vi "Test Basic Forms.vi"() -> ()   [LabVIEW 2020]
uses:
  HTTP Server/Server/Server.lvclass
  HTTP Server/RequestTraceLog/RequestTraceLog.lvclass
  HTTP Server/StandardFileServe/StandardFileServe.lvclass
  C:/dev/IlluminatedG/lv-http-server/HTTP Server/Controller/Controller.lvclass
  C:/dev/IlluminatedG/lv-http-server/HTTP Server/Handler/Handler.lvclass
  C:/dev/IlluminatedG/lv-http-server/HTTP Server/StandardFileServe/StandardFileServe.lvclass
  HTTP Server/Processing Step.ctl
  HTTP Server/HTTP Server.lvlib
  HTTP Server/Trace Item.ctl
  HTTP Server/Trace Log.ctl
panel:
  in  "Debug":bool=TRUE
  out "error out":errorcluster
  in  "Port":u16=36987
  in  "Refresh Traces":bool
  out "Traces":T1[](array[typedef]) {"Items"."Time" format="%.6f"}
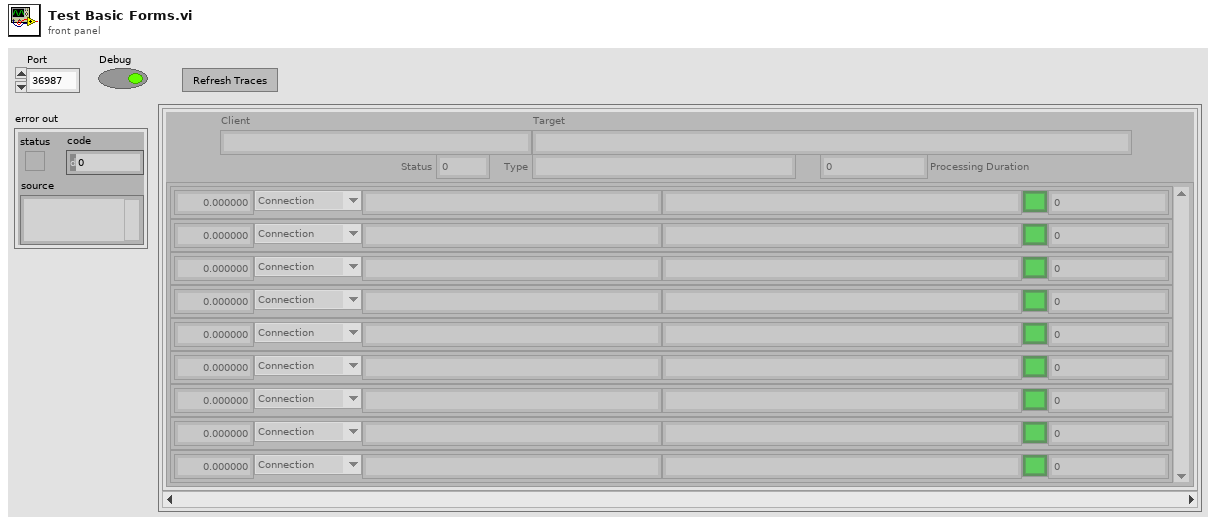
[diagram p1: front panel]
types:
  T1 = typedef "HTTP Server.lvlib/Trace Log.ctl" = cluster{"Client":string, "Target":string, "Status":u16, "Type":string, "Processing Duration":dbl, "Items":T2[]}
  T2 = typedef "HTTP Server.lvlib/Trace Item.ctl" = cluster{"Time":dbl, "Processing Step":T3, "Class":string, "Info":string, "Status":bool, "Code":i32}
  T3 = typedef "HTTP Server.lvlib/Processing Step.ctl" = enum16{"Connection", "Request", "Routing", "Controller Init", "Controller", "Response", "Complete", "Exception"}
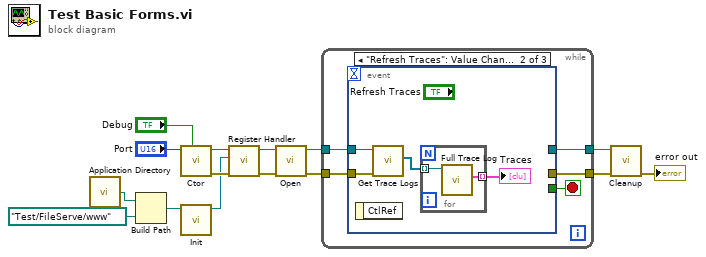
[diagram p0: block diagram]
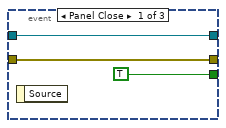
[diagram p2: hidden frame]
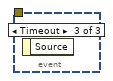
[diagram p3: hidden frame]
diagram:
  n1 = call <vilib>:"Application Directory.vi"() -> ("Application Directory"=w9:path)
  n2 = Build Path(base path=w9, name or relative path=path "Test/FileServe/www") -> (appended path=w7:path)
  n3 = call "Ctor.vi"("Debug (F)"="Debug", "Port (8080)"="Port") -> ("error out"=w3:errorcluster, "Server out"=w5:refnum<class "Server.lvclass">)  [unwired: 8 in]
  n4 = call "Init.vi"("Public Root"=w7) -> ("StandardFileServe out"=w1:refnum<class "StandardFileServe.lvclass">)  [unwired: 9 in, 1 out]
  n5 = call "Register Handler.vi"("error in (no error)"=w3, "Handler"=w1, "Server in"=w5) -> ("error out"=w2:errorcluster, "Server out"=w4:refnum<class "Server.lvclass">)  [unwired: 7 in]
  n6 = call "Open.vi"("error in (no error)"=w2, "Server in"=w4) -> ("error out"=w13:errorcluster, "Server out"=w14:refnum<class "Server.lvclass">)  [unwired: 8 in]
  n7 = while {
    tunnel: w14 -> [w18]
    tunnel: w13 -> [w19]
    tunnel: [w17] -> w12
    tunnel: [w16] -> w11
    stop <- w20 stop-if-true
    n8 = event shown="[1] \"Refresh Traces\": Value Change" {
      selector: _ -> [_ _ _]
      dyn-events: _ -> [_ _ _]
      timeout: _ -> [_ _ _]
      tunnel: [TRUE ("Discard?") _ _] -> w20
      tunnel: w19 -> [w21 w26 _]
      tunnel: w18 -> [w22 w27 _]
      tunnel: [w22 _ _] -> w17
      tunnel: [w21 _ _] -> w16
      event Panel Close {
        n9 = event-data() -> ()  [unwired: 1 in, 1 out]
      }
      event "Refresh Traces": Value Change {
        n10 = event-data() -> ()  [unwired: 1 in, 1 out]
        n11 = call "Get Trace Logs.vi"("error in (no error)"=w26, "Server in"=w27) -> ("Trace Logs"=w25:refnum<class "RequestTraceLog.lvclass">[])  [unwired: 7 in, 2 out]
        n12 = for {
          tunnel: w25 -> [w29] mode=indexing
          tunnel: [w28] -> w24 mode=indexing
          n13 = call "Full Trace Log.vi"("RequestTraceLog in"=w29) -> ("Trace Log"=w28:T1)  [unwired: 8 in, 2 out]
        }
        "Traces" <- w24
      }
      event Timeout {
        n14 = event-data() -> ()  [unwired: 1 in, 1 out]
      }
    }
  }
  n15 = call "Cleanup.vi"("error in (no error)"=w11, "Server in"=w12) -> ("error out"=→"error out":errorcluster)  [unwired: 9 in]
